vi "ReadMsg.vi"(0 "reference in":refnum<class "MessageAMC.lvclass">, 5 "timeout (10 s)":i32=10000, 11 "error in (no error)":errorcluster) -> (3 "exit process?":bool, 4 "reference out":refnum<class "MessageAMC.lvclass">, 6 "message":T1, 8 "timed out?":bool, 15 "error out":errorcluster)   [LabVIEW 2019, in "MessageAMC.lvclass"]
uses:
  MessageAMC.lvclass
  MessageInterface_class/Message.ctl
  MessageAMC.lvclass/MessageAMC.ctl
  <vilib>/NI/AMC/Read Termination Message.vi
  <vilib>/NI/AMC/Create Single Message.vi
  <vilib>/NI/AMC/Globals.vi
  <vilib>/NI/AMC/AMC.lvlib
  MessageInterface_class/MessageInterface.lvclass
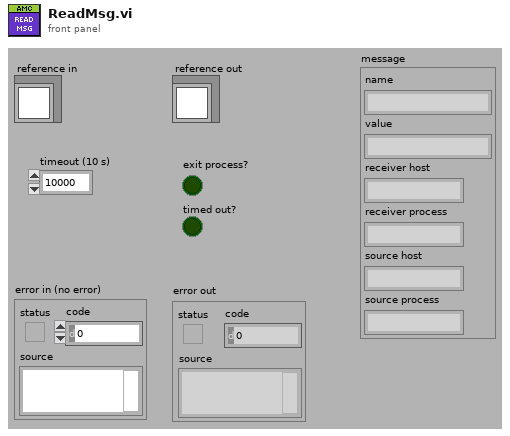
[diagram p1: front panel]
types:
  T1 = typedef "MessageInterface.lvclass/Message.ctl" = cluster{"name":string, "value":string, "receiver host":string, "receiver process":string, "source host":string, "source process":string}
  T2 = typedef "AMC.lvlib/Message Queue.ctl" = refnum<queue>
  T3 = typedef "AMC.lvlib/Message.ctl" = cluster{"name":string, "value":string, "attributes":T4, "receiver host":string, "receiver process":string, "source host":string, "source process":string, "priority message":bool, "acknowledge message":bool}
  T4 = typedef "Tools_KeyedArray.lvlib/KeyedArray.ctl" = cluster{"keys":string[], "values":string[]}
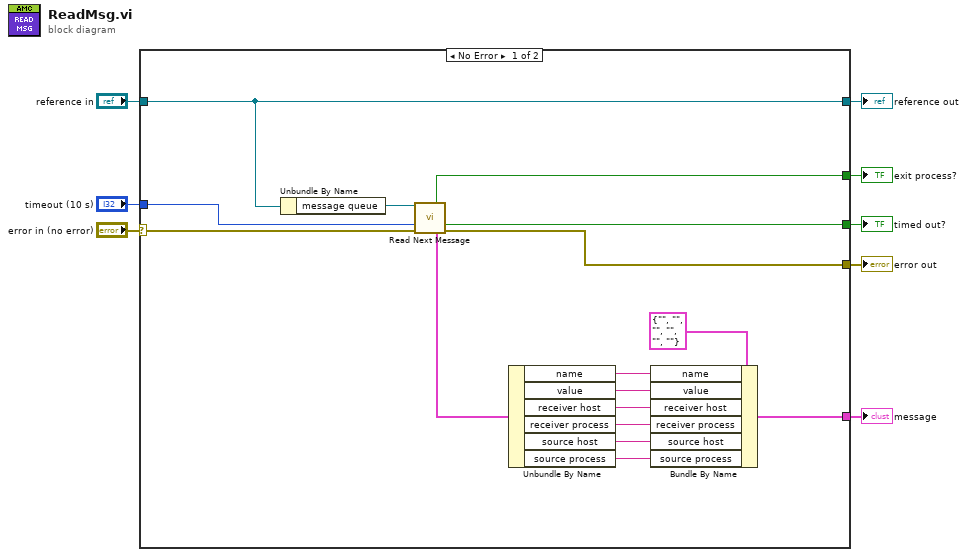
[diagram p0: block diagram]
diagram:
  n1 = case shown="No Error" "error in (no error)" {
    selector: "error in (no error)" -> [w24 w26]
    tunnel: [w20 w26] -> w7
    tunnel: [w23 w25] -> w5
    tunnel: "reference in" -> [w23 w25]
    tunnel: "timeout (10 s)" -> [w21 _]
    tunnel: [w17 _] -> w1
    tunnel: [w19 _] -> w3
    tunnel: [w18 _] -> w2
    frame No Error {
      n2 = Unbundle By Name(w23) -> ("message queue"=w22:T2)
      n3 = call <vilib>:"Read Next Message.vi"("message queue in"=w22, "timeout (1 ms)"=w21, "error in"=w24) -> ("exit process?"=w19:bool, "timed out?"=w18:bool, "message"=w16:T3, "error out"=w20:errorcluster)  [unwired: 5 in, 4 out]
      n4 = Unbundle By Name(w16) -> ("name"=w15:string, "value"=w14:string, "receiver host"=w12:string, "receiver process"=w11:string, "source host"=w10:string, "source process"=w9:string)
      n5 = Bundle By Name(cluster=T1 {"name"="", "value"="", "receiver host"="", "receiver process"="", "source host"="", "source process"=""} ("message"), "name"=w15, "value"=w14, "receiver host"=w12, "receiver process"=w11, "source host"=w10, "source process"=w9) -> (w17:T1)
    }
    frame Error {
    }
  }
  "error out" <- w7
  "reference out" <- w5
  "exit process?" <- w3
  "timed out?" <- w2
  "message" <- w1
